vi "GUI_Smaract_v1.0.0.vi"() -> ()   [LabVIEW 2013]
uses:
  Shared/Device Driver/OnOffTypeDef.ctl
panel:
  out "indecator ref array":refnum<vi>[](array[refnum])
  in  "time to wait (TCP) 2":i32=10
  in  "plot":bool=TRUE
  out "ratio(h)":bool
  out "fixsize":bool
  in  "shotnumber":i32
  out "error (h)":bool
  out "Device Name (h)":string="StagingDG645 1"
  in  "Main Tap":T1(tab)
  in  "Home.Channel 1":T2
  out "InternalStatus.Channel 2":T3(ring)
  in  "ReferencePosition.Channel 2":dbl format="%#_10f"
  in  "filter.Channel 2":T2
  in  "Position.Channel 2":dbl format="%#_10f"
  in  "ReferencePosition.Channel 1":dbl format="%#_10f"
  in  "Position.Channel 1":dbl format="%#_10f"
  in  "filter.Channel 1":T2
  in  "DBasReferenceSource":T2
  out "InternalStatus.Channel 1":T3(ring)
  out "local Port":u16=65427
  out "port or service name":u16=65426
  out "Remote Host":string="192.168.11.97"
  in  "timeout ms (slow resp)":i32=500
  in  "reset":bool
  out "image con closed":bool
  out "image \nconnection":bool
  out "image con closed 2":bool=TRUE
  out "All Devices (h)":string[](array[string])=["StagingDG645 1", "StagingDG645 2"]
  in  "time to wait (TCP)":i32=10
  out "error out":errorcluster
  out "connections (hidden)":variant[](array[variant])=[variant(refnum<k16> refnum), variant(refnum<k16> refnum)]
  in  "time to wait (main loop)":i32=10
  out "Data String":string="Amplitude.Ch AB,3.000000000000\r\nAmplitude.Ch CD,4.000000000000\r\nAmplitude.Ch EF,4.000000000000\r\nAmplitude.Ch GH,4.000000000000\r\nAmplitude.Ch T0,4.000000000000\r\nDelay.Ch A,0.000000000000\r\nDelay.Ch B,0.030000000000\r\nDelay.Ch C,0.000000000000\r\nDelay.Ch D,0.030000000000\r\nDelay.Ch E,0.000000000000\r\nDelay.Ch F,0.030000000000\r\nDelay.Ch G,0.000000000000\r\nDelay.Ch H,0.030000000000\r\nDelay.Ch T0,0.000000000000\r\nDelay.Ch T1,0.030000\r\nInhibit,Triggers\r\nLinked.Ch A,T0\r\nLinked.Ch B,A\r\nLinked.Ch C,T0\r\nLinked.Ch D,C\r\nLinked.Ch E,T0\r\nLinked.Ch F,E\r\nLinked.Ch G,T0\r\nLinked.Ch H,G\r\nLocalSavingPath,c:\\temp\r\nSave,off\r\nTrigger.ExecuteSingleShot,\r\nTrigger.Level,1.000000\r\nTrigger.Rate,10.000000\r\nTrigger.Source,External rising edges\r\ntimeout,0.000000\r\nPolarity.Ch AB,Positive\r\nPolarity.Ch CD,Positive\r\nPolarity.Ch EF,Positive\r\nPolarity.Ch GH,Positive\r\nPolarity.Ch T0,Positive\r\n"
  in  "Local Saving Path":path
  out "String":string
  out "error message":string
  out "Data Connection out":bool=TRUE
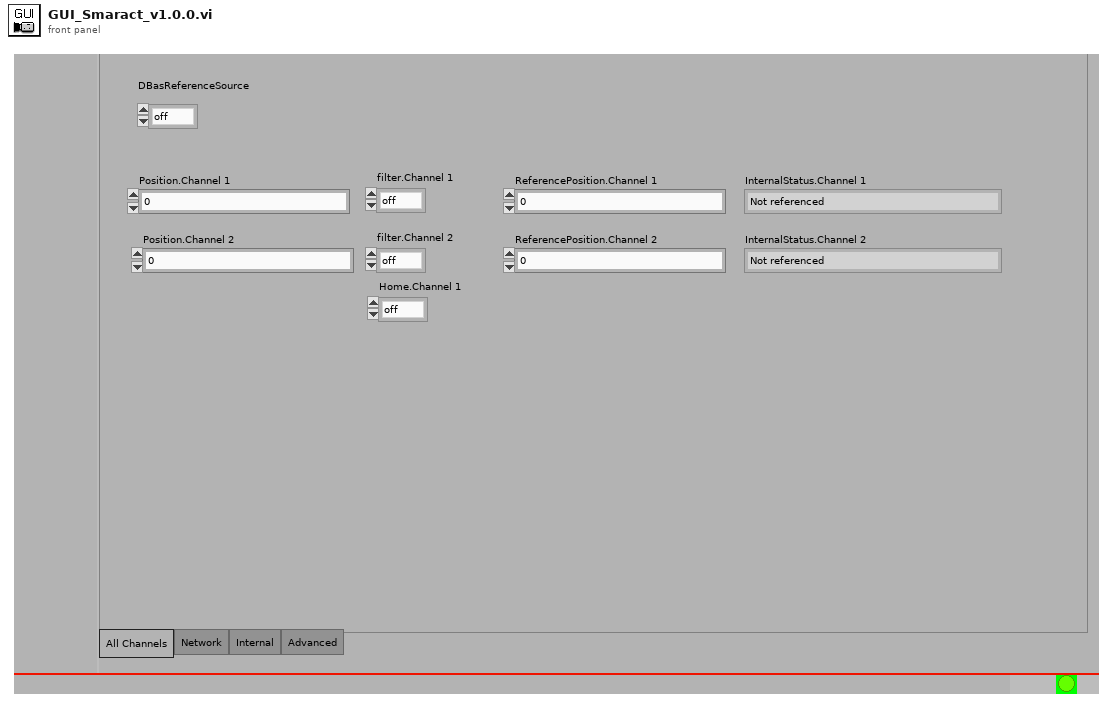
[diagram p1: front panel]
types:
  T1 = enum32{"All Channels", "Network", "Internal", "Advanced"}
  T2 = typedef "OnOffTypeDef.ctl" = enum16{"off", "on"}
  T3 = enum16{"Not referenced", "Homing", "Moving", "Ready"}
  T4 = typedef "EventTypDef.ctl" = refnum<user-event>
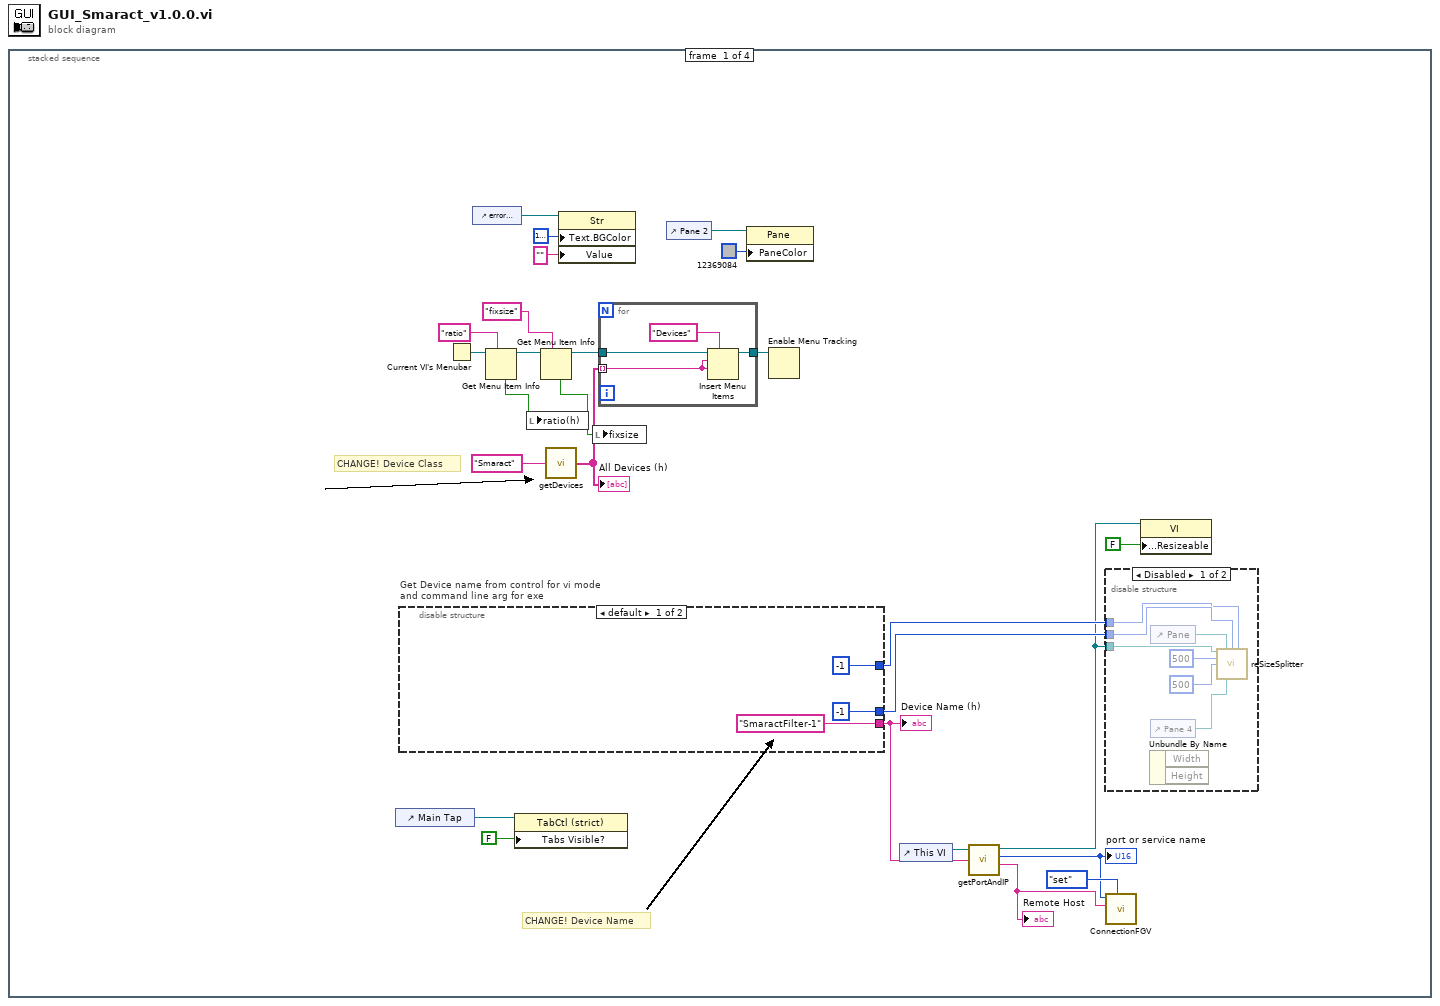
[diagram p0: block diagram]
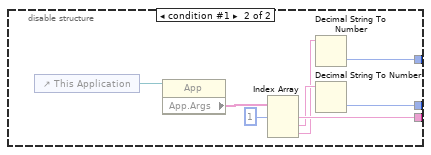
[diagram p3: hidden frame]
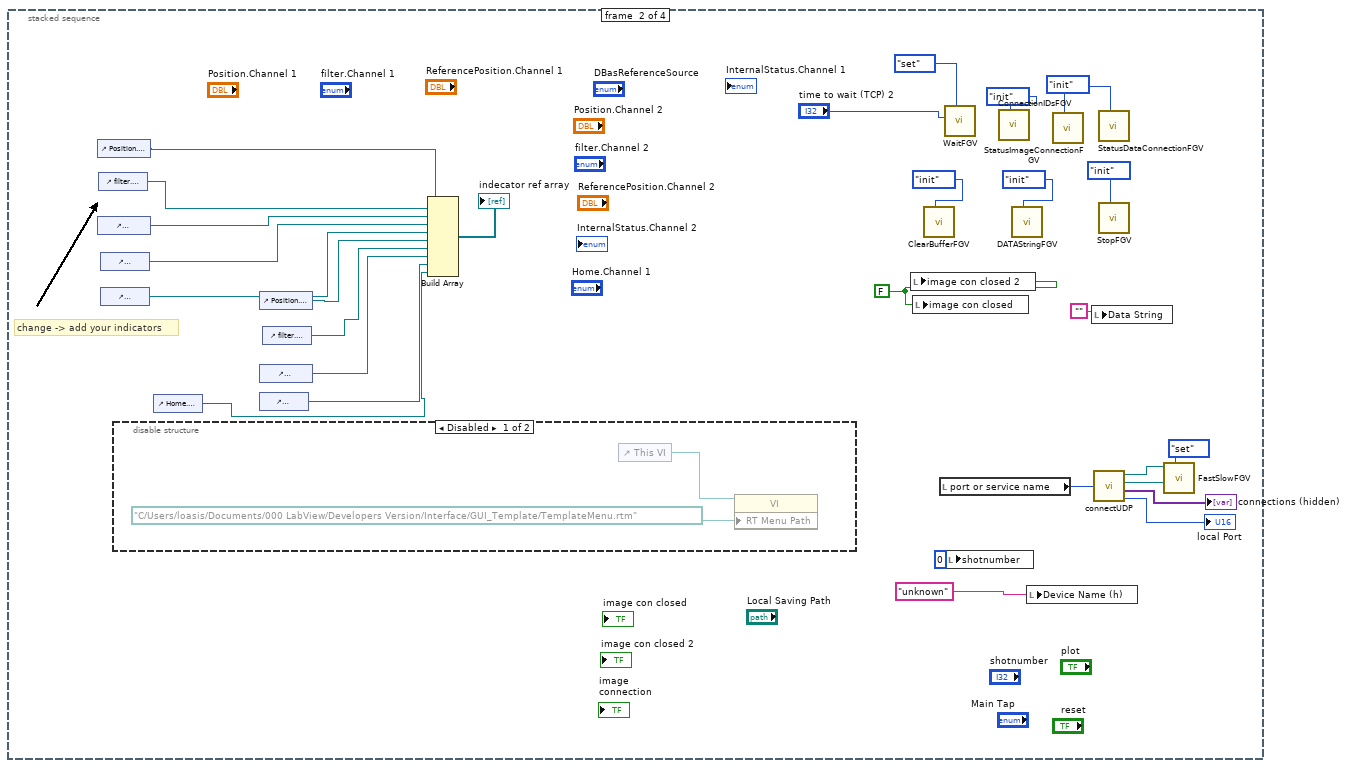
[diagram p4: hidden frame]
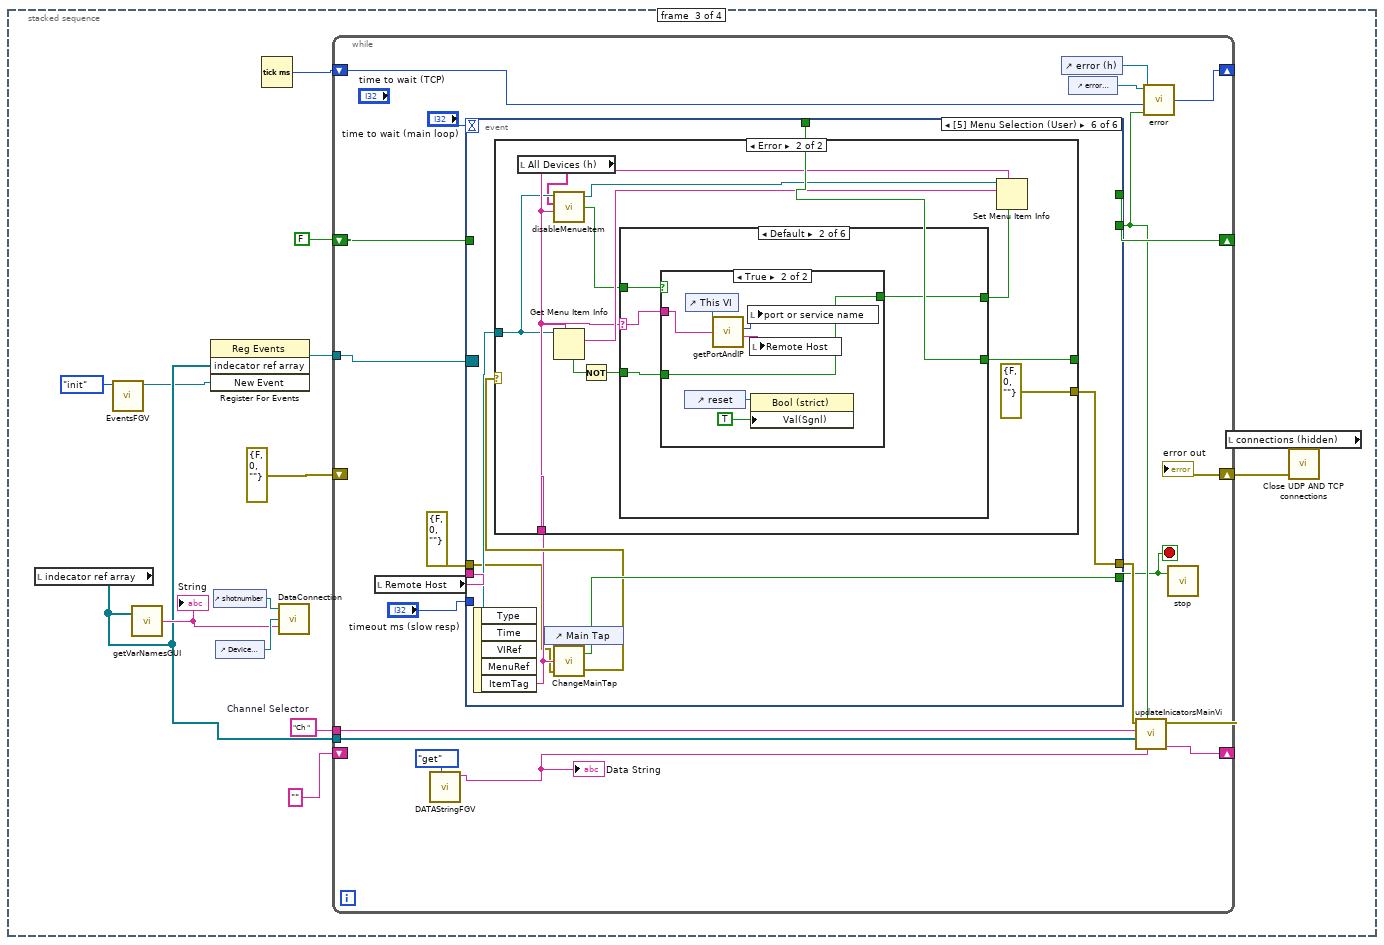
[diagram p6: hidden frame]
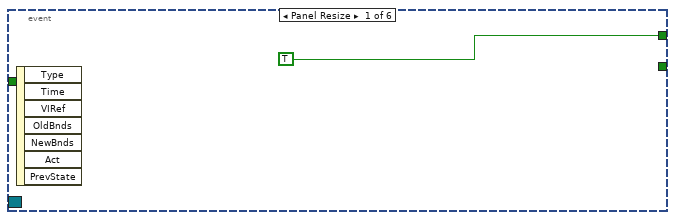
[diagram p7: hidden frame]
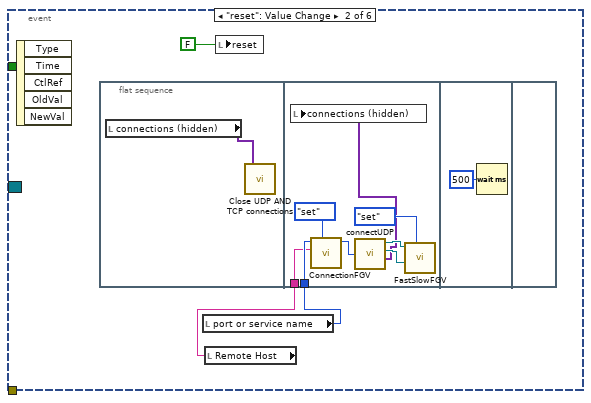
[diagram p8: hidden frame]
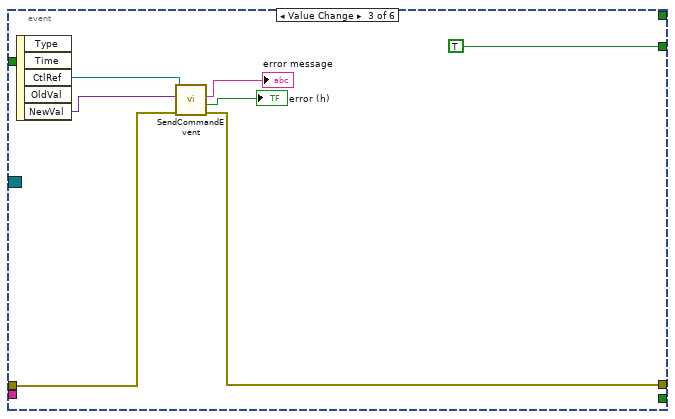
[diagram p9: hidden frame]
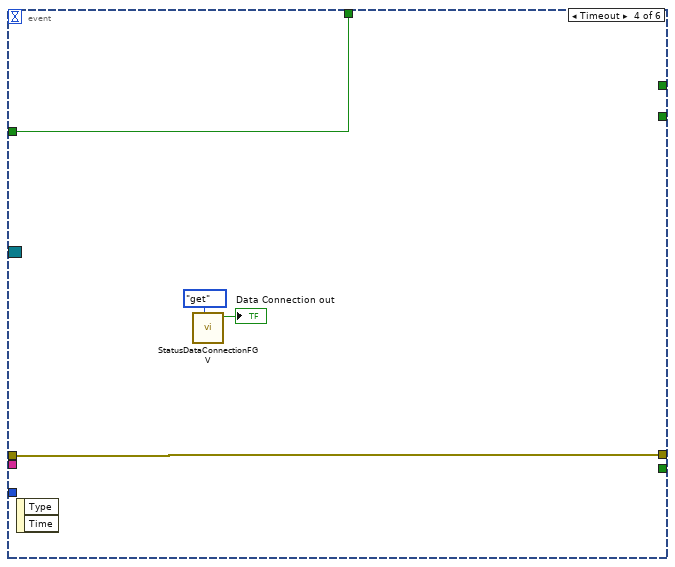
[diagram p10: hidden frame]
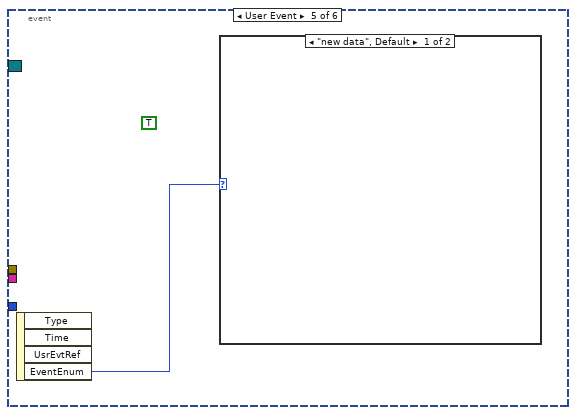
[diagram p11: hidden frame]
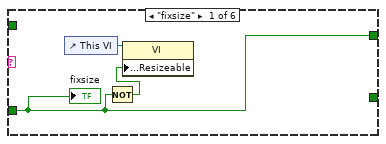
[diagram p14: hidden frame]
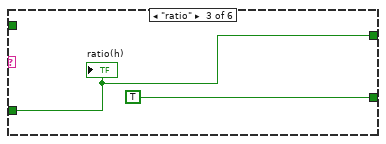
[diagram p16: hidden frame]
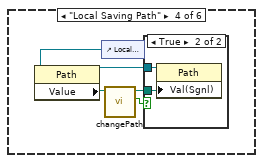
[diagram p17: hidden frame]
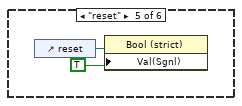
[diagram p19: hidden frame]
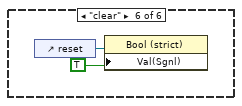
[diagram p20: hidden frame]
diagram:
  n1 = stacked-sequence {
    frame #0 {
      # "CHANGE! Device Name"
      # "CHANGE! Device Class"
      n2 = control-ref of="Main Tap"() -> (w26:refnum<vi>)
      n3 = disable-structure "Get Device name from control for vi mode\nand command line arg for exe" shown="default" {
        disable-tunnel: ["SmaractFilter-1" ("Device Name for vi mode") w45] -> w22
        disable-tunnel: [i16 -1 ("left") w42] -> w24
        disable-tunnel: [i16 -1 ("left") w41] -> w23
        frame condition #0 (active) {
        }
        frame condition #1 {
          n4 = control-ref of="This Application"() -> (w48:refnum<vi>)
          n5 = property class="App"(reference=w48) -> ("App.Args"=w47:string[])  [unwired: 1 in, 2 out]
          n6 = Index Array(array=w47, index #1=1 ("index")) -> (element #1=w45:string, element #2=w44:string, element #3=w43:string)  [unwired: 2 in]
          n7 = Decimal String To Number(string=w43) -> (number=w41:i32)  [unwired: 2 in, 1 out]
          n8 = Decimal String To Number(string=w44) -> (number=w42:i32)  [unwired: 2 in, 1 out]
        }
      }
      "Device Name (h)" <- w22
      n9 = Current VI's Menubar() -> (w14:refnum<k9>)
      n10 = control-ref of="error message"() -> (w8:refnum<vi>)
      n11 = Get Menu Item Info(7:"ratio" ("item tag"), 11:w14) -> (3:w12:refnum<k9>, 4:w13:bool)  [unwired: 1 in, 5 out]
      n12 = property class="TabCtl (strict)"(reference=w26, "Tabs Visible?"=FALSE) -> ()  [unwired: 1 in, 2 out]
      n13 = local write "ratio(h)"(w13) -> ()
      n14 = Get Menu Item Info(7:"fixsize" ("item tag"), 11:w12) -> (3:w4:refnum<k9>, 4:w10:bool)  [unwired: 1 in, 5 out]
      n15 = call "getDevices.vi"("Device Class"="Smaract") -> ("All Devices"=w2:string[])
      "All Devices (h)" <- w2
      n16 = property class="Str"(reference=w8, "Text.BGColor"=u32 16777238, "Value"="") -> ()  [unwired: 1 in, 2 out]
      n17 = local write "fixsize"(w10) -> ()
      n18 = for {
        tunnel: w4 -> [w30]
        tunnel: [w29] -> w3
        tunnel: w2 -> [w27] mode=indexing
        n19 = Insert Menu Items(5:"Devices" ("menu tag"), 7:w27, 8:w27, 9:w30) -> (3:w29:refnum<k9>)  [unwired: 2 in, 2 out]
      }
      n20 = control-ref of="Pane 2"() -> (w6:refnum<vi>)
      n21 = property class="Pane"(reference=w6, "PaneColor"=u32 12369084) -> ()  [unwired: 1 in, 2 out]
      n22 = Enable Menu Tracking(4:w3) -> ()  [unwired: 2 in, 2 out]
      n23 = control-ref of="This VI"() -> (w21:refnum<vi>)
      n24 = call "getPortAndIP.vi"("Device Name"=w22, "This Vi"=w21) -> ("Remote Host"=w17:string, "port or service name"=w16:u16, "reference out"=w19:refnum<vi>)  [unwired: 2 in, 2 out]
      "port or service name" <- w16
      "Remote Host" <- w17
      n25 = disable-structure shown="Disabled" {
        disable-tunnel: w24 -> [w36 _]
        disable-tunnel: w23 -> [w35 _]
        disable-tunnel: w19 -> [w33 _]
        frame Disabled {
          n26 = Unbundle By Name() -> ()  [unwired: 1 in, 2 out]
          n27 = control-ref of="Pane"() -> (w37:refnum<vi>)
          n28 = control-ref of="Pane 4"() -> (w34:refnum<vi>)
          n29 = call "reSizeSplitter.vi"("this vi"=w33, "pane"=w37, "left"=w36, "top"=w35, "Width"=u32 500, "Height"=u32 500, "pane2"=w34) -> ()  [unwired: 8 in, 1 out]
        }
        frame Enabled {
        }
      }
      n30 = call "ConnectionFGV.vi"("command"=enum16{"get", "set", "init"}."set", "Remote Host in"=w17, "port or service name in"=w16) -> ()  [unwired: 7 in, 2 out]
      n31 = property class="VI"(reference=w19, "Front Panel.Resizeable"=FALSE ("Front Panel Window:Resizable")) -> ()  [unwired: 1 in, 2 out]
    }
    frame #1 {
      w68 = enum16{"get", "set", "init"}."init" ("Command")
      w74 = FALSE ("new Device Data")
      # "change -> add your indicators"
      n32 = control-ref of="Position.Channel 1"() -> (w58:refnum<vi>)
      n33 = control-ref of="ReferencePosition.Channel 1"() -> (w56:refnum<vi>)
      n34 = control-ref of="filter.Channel 1"() -> (w57:refnum<vi>)
      n35 = control-ref of="DBasReferencePosition"() -> (w55:refnum<vi>)
      n36 = control-ref of="InternalStatus.Channel 1"() -> (w54:refnum<vi>)
      n37 = disable-structure shown="Disabled" {
        frame Disabled {
          n38 = control-ref of="This VI"() -> (w78:refnum<vi>)
          n39 = property class="VI"(reference=w78, "RT Menu Path"=path "C:/Users/loasis/Documents/000 LabView/Developers Version/Interface/GUI_Template/TemplateMenu.rtm" ("Run-Time Menu Path")) -> ()  [unwired: 1 in, 2 out]
        }
        frame Enabled {
        }
      }
      n40 = control-ref of="Home.Channel 1"() -> (w49:refnum<vi>)
      n41 = control-ref of="Position.Channel 2"() -> (w53:refnum<vi>)
      n42 = control-ref of="ReferencePosition.Channel 2"() -> (w51:refnum<vi>)
      n43 = control-ref of="InternalStatus.Channel 2"() -> (w50:refnum<vi>)
      n44 = control-ref of="filter.Channel 2"() -> (w52:refnum<vi>)
      n45 = Build Array(w58, w57, w56, w55, w54, w53, w52, w51, w50, w49) -> (→"indecator ref array":refnum<vi>[])
      n46 = local write "image con closed 2"(w74) -> ()
      n47 = local write "image con closed"(w74) -> ()
      n48 = call "ClearBufferFGV.vi"("Command"=enum16{"set", "get", "init"}."init") -> ()  [unwired: 10 in, 1 out]
      n49 = local read "port or service name"() -> (w64:u16)
      n50 = call "WaitFGV.vi"("Command"=enum16{"get", "set", "init"}."set", "milliseconds to wait"="time to wait (TCP) 2") -> ()  [unwired: 9 in, 1 out]
      n51 = local write "shotnumber"(0 ("shotnumber")) -> ()
      n52 = call "ConnectionIDsFGV.vi"("Command"=enum16{"add", "get", "init"}."init") -> ()  [unwired: 10 in, 1 out]
      n53 = call "DATAStringFGV.vi"("Command"=enum16{"get", "set", "init"}."init") -> ()  [unwired: 9 in, 2 out]
      n54 = local write "Device Name (h)"("unknown" ("Device Name")) -> ()
      n55 = call "StatusImageConnectionFGV.vi"("Command"=w68) -> ()  [unwired: 10 in, 1 out]
      n56 = local write "Data String"("") -> ()
      n57 = call "connectUDP.vi"("port or service name NOT USED"=w64) -> ("fast ID (h)"=w63:refnum<k16>, "slow ID (h)"=w62:refnum<k16>, "connections (hidden)"=→"connections (hidden)":variant[], "local Port"=→"local Port":u16)
      n58 = call "StatusDataConnectionFGV.vi"("Command"=w68) -> ()  [unwired: 10 in, 1 out]
      n59 = call "StopFGV.vi"("Command"=enum16{"set", "get", "init"}."init") -> ()  [unwired: 9 in, 2 out]
      n60 = call "FastSlowFGV.vi"("Command"=enum16{"get", "set", "init"}."set", "slow ID"=w62, "fast ID"=w63) -> ()  [unwired: 7 in, 2 out]
    }
    frame #2 {
      w83 = "Ch "  # Channel Selector
      n61 = local read "indecator ref array"() -> (w81:refnum<vi>[])
      n62 = call "EventsFGV.vi"("Command"=enum16{"get", "init"}."init") -> ("New Event"=w79:T4)  [unwired: 9 in, 1 out]
      n63 = call "getVarNamesGUI.vi"("Array"=w81) -> ("String"=w82:string)  [unwired: 1 in]
      "String" <- w82
      n64 = register-events(w81, w79) -> (reference out=w84:refnum<event-registration>)  [unwired: 2 in, 1 out]
      n65 = control-ref of="shotnumber"() -> (w86:refnum<vi>)
      n66 = control-ref of="Device Name (h)"() -> (w85:refnum<vi>)
      n67 = Tick Count (ms)() -> (millisecond timer value=w88:u32)
      n68 = call "DataConnection.vi"("Subscriber list"=w82, "Device Name (h)"=w85, "shotnumber"=w86) -> ()
      n69 = while {
        shift-right: [w108] -> w91
        shift-left: errorcluster {"status"=FALSE, "code"=0, "source"=""} ("error out") -> [_]
        tunnel: w81 -> [w102]
        shift-right: [w106] -> _
        shift-left: FALSE -> [w107]
        shift-right: [w105] -> _
        shift-left: w88 -> [w104]
        shift-right: [w95] -> _
        shift-left: "" ("Data String") -> [_]
        tunnel: w84 -> [w98]
        tunnel: w83 -> [w97]
        stop <- w99 stop-if-true
        n70 = local read "Remote Host"() -> (w110:string)
        n71 = call "DATAStringFGV.vi"("Command"=enum16{"get", "set", "init"}."get") -> ("Data String out"=w100:string)  [unwired: 9 in, 1 out]
        "Data String" <- w100
        n72 = event shown="[5] Menu Selection (User)" {
          selector: w98 -> [_ _ _ _ _ _]
          dyn-events: _ -> [_ _ _ _ _ _]
          timeout: "time to wait (main loop)" -> [_ _ _ _ _ _]
          tunnel: [_ _ w131 w137 _ w140] -> w109
          tunnel: w110 -> [_ _ _ _ _ _]
          tunnel: "timeout ms (slow resp)" -> [_ _ _ _ _ _]
          tunnel: errorcluster {"status"=FALSE, "code"=0, "source"=""} ("error out") -> [_ _ w128 w137 _ w141]
          tunnel: [_ _ TRUE _ _ _] -> w103
          tunnel: [_ _ _ _ _ w146] -> w99
          tunnel: [_ _ _ w136 _ w143] -> _
          tunnel: w107 -> [_ _ _ w136 _ _]
          tunnel: [TRUE _ _ _ _ _] -> w106
          event Panel Resize {
            n73 = event-data() -> ()  [unwired: 1 in, 7 out]
          }
          event "reset": Value Change {
            n74 = event-data() -> ()  [unwired: 1 in, 5 out]
            n75 = flat-sequence {
              tunnel: w115 -> [w120]
              tunnel: w114 -> [w119]
              frame #0 {
                n76 = local read "connections (hidden)"() -> (w117:variant[])
                n77 = call "Close UDP AND TCP connections.vi"("appended array"=w117) -> ()  [unwired: 7 in]
              }
              frame #1 {
                n78 = call "ConnectionFGV.vi"("command"=enum16{"get", "set", "init"}."set", "Remote Host in"=w119, "port or service name in"=w120) -> ("port or service name out"=w124:u16)  [unwired: 7 in, 1 out]
                n79 = call "connectUDP.vi"("port or service name NOT USED"=w124) -> ("fast ID (h)"=w123:refnum<k16>, "slow ID (h)"=w122:refnum<k16>, "connections (hidden)"=w118:variant[])  [unwired: 1 out]
                n80 = local write "connections (hidden)"(w118) -> ()
                n81 = call "FastSlowFGV.vi"("Command"=enum16{"get", "set", "init"}."set", "slow ID"=w122, "fast ID"=w123) -> ()  [unwired: 7 in, 2 out]
              }
              frame #2 {
                n82 = Wait (ms)(milliseconds to wait=u32 500) -> ()  [unwired: 1 out]
              }
              frame #3 {
              }
            }
            n83 = local read "port or service name"() -> (w115:u16)
            n84 = local read "Remote Host"() -> (w114:string)
            n85 = local write "reset"(FALSE ("reset")) -> ()
          }
          event Value Change {
            n86 = event-data() -> ("CtlRef"=w133:refnum<vi>, "NewVal"=w132:variant)  [unwired: 1 in, 3 out]
            n87 = call "SendCommandEvent.vi"("error out 2"=w128, "NewVal"=w132, "CtlRef"=w133) -> ("error out"=w131:errorcluster, "error (h)"=→"error (h)":bool, "error message"=→"error message":string)  [unwired: 5 in, 1 out]
          }
          event Timeout {
            n88 = event-data() -> ()  [unwired: 1 in, 2 out]
            n89 = call "StatusDataConnectionFGV.vi"("Command"=enum16{"get", "set", "init"}."get") -> ("Data Connection out"=→"Data Connection out":bool)  [unwired: 10 in]
          }
          event User Event {
            (unwired) TRUE
            n90 = event-data() -> ("EventEnum"=w138:enum16{"new data", "connection status update"})  [unwired: 1 in, 3 out]
            n91 = case shown="\"new data\", Default" w138 {
              frame "new data", Default {
              }
              frame "connection status update" {
              }
            }
          }
          event Menu Selection (User) {
            n92 = event-data() -> ("MenuRef"=w142:refnum<k9>, "ItemTag"=w144:string)  [unwired: 1 in, 3 out]
            n93 = control-ref of="Main Tap"() -> (w139:refnum<vi>)
            n94 = call "ChangeMainTap.vi"("error in"=w141, "ItemTag"=w144, "reference"=w139) -> ("error out"=w145:errorcluster, "Boolean"=w146:bool)
            n95 = case shown="Error" w145 {
              selector: w145 -> [w147 _]
              tunnel: w142 -> [_ w153]
              tunnel: [_ w155] -> w143
              tunnel: w144 -> [_ w154]
              tunnel: [w147 errorcluster {"status"=FALSE, "code"=0, "source"=""} ("error IO")] -> w140
              frame No Error {
              }
              frame Error {
                n96 = local read "All Devices (h)"() -> (w148:string[])
                n97 = call "disableMenueItem.vi"("ItemTag"=w154, "All Devices (h)"=w148, "MenuRef"=w153) -> ("this is a Device(tag)"=w152:bool, "menu reference out"=w151:refnum<k9>)  [unwired: 1 in, 1 out]
                n98 = Get Menu Item Info(7:w154, 11:w153) -> (2:w157:string, 4:w158:bool)  [unwired: 1 in, 5 out]
                n99 = Not(x=w158) -> (.not. x?=w156:bool)
                n100 = case shown="Default" w154 {
                  selector: w154 -> [_ w164 _ _ _ _]
                  tunnel: w156 -> [w159 w162 w173 _ _ _]
                  tunnel: [_ _ TRUE _ _ _] -> w155
                  tunnel: w152 -> [_ w165 _ _ _ _]
                  tunnel: [w159 w163 w173 _ _ _] -> w150
                  frame "fixsize" {
                    n101 = control-ref of="This VI"() -> (w161:refnum<vi>)
                    n102 = Not(x=w159) -> (.not. x?=w160:bool)
                    n103 = property class="VI"(reference=w161, "Front Panel.Resizeable"=w160) -> ()  [unwired: 1 in, 2 out]
                    "fixsize" <- w159
                  }
                  frame Default {
                    n104 = case shown="True" w165 {
                      tunnel: w164 -> [_ w172]
                      tunnel: [_ w166] -> w163
                      tunnel: w162 -> [_ w166]
                      frame False {
                      }
                      frame True {
                        n105 = control-ref of="reset"() -> (w168:refnum<vi>)
                        n106 = control-ref of="This VI"() -> (w171:refnum<vi>)
                        n107 = call "getPortAndIP.vi"("Device Name"=w172, "This Vi"=w171) -> ("Remote Host"=w170:string, "port or service name"=w169:u16)  [unwired: 2 in, 3 out]
                        n108 = local write "port or service name"(w169) -> ()
                        n109 = local write "Remote Host"(w170) -> ()
                        n110 = property class="Bool (strict)"(reference=w168, "Val(Sgnl)"=TRUE ("Value (Signaling)")) -> ()  [unwired: 1 in, 2 out]
                      }
                    }
                  }
                  frame "ratio" {
                    "ratio(h)" <- w173
                  }
                  frame "Local Saving Path" {
                    n111 = control-ref of="Local Saving Path"() -> (w175:refnum<vi>)
                    n112 = property class="Path"(reference=w175) -> (reference out=w178:refnum<vi>, "Value"=w179:path)  [unwired: 1 in, 1 out]
                    n113 = call "changePath.vi"("Local Saving in (h)"=w179) -> ("change (h)"=w177:bool, "Local Saving out (h)"=w176:path)  [unwired: 9 in]
                    n114 = case shown="True" w177 {
                      tunnel: w178 -> [_ w181]
                      tunnel: w176 -> [_ w180]
                      frame False {
                      }
                      frame True {
                        n115 = property class="Path"(reference=w181, "Val(Sgnl)"=w180) -> ()  [unwired: 1 in, 2 out]
                      }
                    }
                  }
                  frame "reset" {
                    n116 = control-ref of="reset"() -> (w183:refnum<vi>)
                    n117 = property class="Bool (strict)"(reference=w183, "Val(Sgnl)"=TRUE ("Value (Signaling)")) -> ()  [unwired: 1 in, 2 out]
                  }
                  frame "clear" {
                    n118 = control-ref of="reset"() -> (w185:refnum<vi>)
                    n119 = property class="Bool (strict)"(reference=w185, "Val(Sgnl)"=TRUE ("Value (Signaling)")) -> ()  [unwired: 1 in, 2 out]
                  }
                }
                n120 = Set Menu Item Info(6:w150, 7:w154, 10:w157, 11:w151) -> ()  [unwired: 3 in, 2 out]
              }
            }
          }
        }
        n121 = control-ref of="error (h)"() -> (w93:refnum<vi>)
        n122 = control-ref of="error message"() -> (w94:refnum<vi>)
        n123 = call "updateInicatorsMainVi.vi"("Data String out"=w100, "Boolean"=w103, "Array"=w102, "Channel Selector"=w97, "error in"=w109) -> ("Data String out 2"=w95:string, "error out"=w108:errorcluster)  [unwired: 4 in, 1 out]
        "error out" <- w108
        n124 = call "error.vi"("Boolean"=w103, "millisecond timer value"=w104, "reference"=w93, "error message"=w94) -> ("millisecond timer value 2"=w105:u32)
        n125 = call "stop.vi"("Boolean"=w99) -> ()
      }
      n126 = local read "connections (hidden)"() -> (w90:variant[])
      n127 = call "Close UDP AND TCP connections.vi"("error in"=w91, "appended array"=w90) -> ()  [unwired: 6 in]
    }
    frame #3 {
      n128 = control-ref of="Main  Control"() -> (w187:refnum<vi>)
      n129 = property class="TabCtl (strict)"(reference=w187, "Tabs Visible?"=TRUE) -> ()  [unwired: 1 in, 2 out]
      n130 = property class="TabCtl (strict)"(reference=w187, "Tab Location"=enum32{"Top", "Bottom", "Left", "Right"}."Bottom") -> ()  [unwired: 1 in, 2 out]
      n131 = flat-sequence {
        frame #0 {
          n132 = Wait (ms)(milliseconds to wait=u32 0) -> ()  [unwired: 1 out]
        }
        frame #1 {
        }
        frame #2 {
          n133 = control-ref of="This VI"() -> (w192:refnum<vi>)
          n134 = case shown="True" FALSE {
            tunnel: w192 -> [w193 w196]
            tunnel: [w193 w194] -> w191
            frame False {
            }
            frame True {
              n135 = property class="VI" props=["Front Panel.Open"](reference=w196) -> (reference out=w195:refnum<vi>)  [unwired: 1 in, 2 out]
              n136 = invoke class="VI" method="FP.Close"(reference=w195) -> (reference out=w194:refnum<vi>)  [unwired: 2 in, 2 out]
            }
          }
          n137 = Close Reference(reference=w191) -> ()  [unwired: 1 in, 1 out]
        }
      }
    }
  }
